vi "Acquire.vi"(8 "error in (no error)":cluster{"状态":bool, "代码":i32, "源":string} caption="错误输入（无错误）", 9 "数据队列":refnum<queue>, 10 "数据通知器":refnum<notifier>, 11 "硬件资源输入":T1) -> (0 "error out":cluster{"状态":bool, "代码":i32, "源":string} caption="错误输出", 3 "硬件资源输出":T1)   [LabVIEW 2014, in "Acquisition.lvlib"]
doc: "执行采集。替换程序框图的内容，添加对采集硬件的调用。"
uses:
  Acquisition.lvlib
  Hardware Configuration.ctl
  Signal Type.ctl
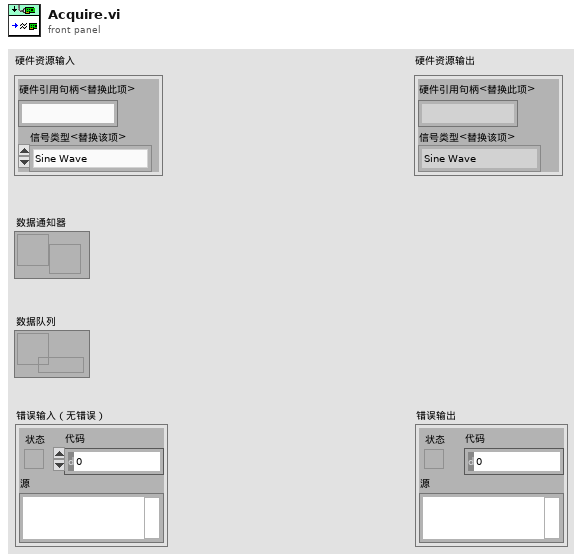
[diagram p1: front panel]
types:
  T1 = typedef "Acquisition.lvlib/Hardware Configuration.ctl" = cluster{"硬件引用句柄<替换此项>":string, "信号类型<替换该项>":T2}
  T2 = typedef "Acquisition.lvlib/Signal Type.ctl" = enum16{"Sine Wave", "Square with Noise"}
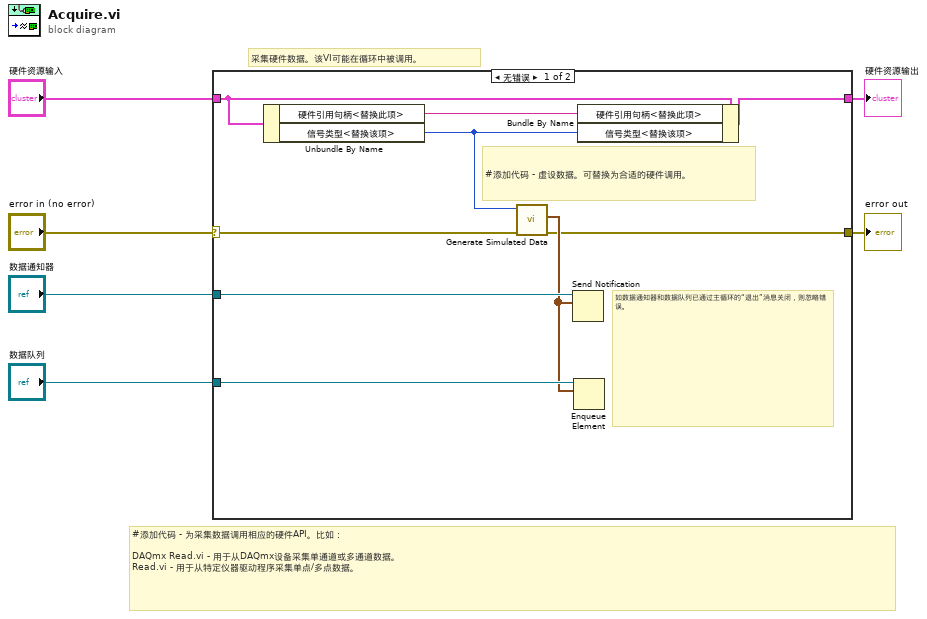
[diagram p0: block diagram]
diagram:
  # "采集硬件数据。该VI可能在循环中被调用。"
  # "#添加代码 - 为采集数据调用相应的硬件API。比如：\n\nDAQmx Read.vi - 用于从DAQmx设备采集单通道或多通道数据。\nRead.vi - 用于从特定仪器驱动程序采集单点/多点数据。"
  n1 = case shown="无错误" "error in (no error)" {
    selector: "error in (no error)" -> [w14 w16]
    tunnel: [w7 w16] -> w5
    tunnel: "硬件资源输入" -> [w11 w17]
    tunnel: [w15 w17] -> w3
    tunnel: "数据通知器" -> [w10 _]
    tunnel: "数据队列" -> [w9 _]
    frame No Error {
      # "如数据通知器和数据队列已通过主循环的“退出”消息关闭，则忽略错误。"
      # "#添加代码 - 虚设数据。可替换为合适的硬件调用。"
      n2 = Unbundle By Name(w11) -> ("硬件引用句柄<替换此项>"=w12:string, "信号类型<替换该项>"=w13:T2)
      n3 = call "Generate Simulated Data.vi"("error in (no error)"=w14, "信号类型"=w13) -> ("error out"=w7:cluster{"状态":bool, "代码":i32, "源":string}, "图形数据"=w8:waveform(dbl)[])  [unwired: 8 in]
      n4 = Send Notification(notification=w8, notifier=w10) -> ()  [unwired: 1 in, 2 out]
      n5 = Enqueue Element(queue=w9, element=w8) -> ()  [unwired: 2 in, 3 out]
      n6 = Bundle By Name(cluster=w11, "硬件引用句柄<替换此项>"=w12, "信号类型<替换该项>"=w13) -> (w15:T1)
    }
    frame Error {
    }
  }
  "硬件资源输出" <- w3
  "error out" <- w5
